vi "second gate increment fake.vi"(10 "Increment":dbl, 11 "Gate Voltage":dbl) -> ()   [LabVIEW 2021]
panel:
  in  "Voltage Safety Limit":dbl
  # "Second Gate\n Increment"
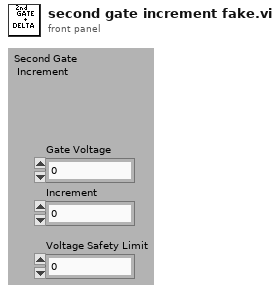
[diagram p1: front panel]
types:
  T1 = enum16{"Set Voltage", "Read Voltage", "Read Current", "Output On", "Output Off"}
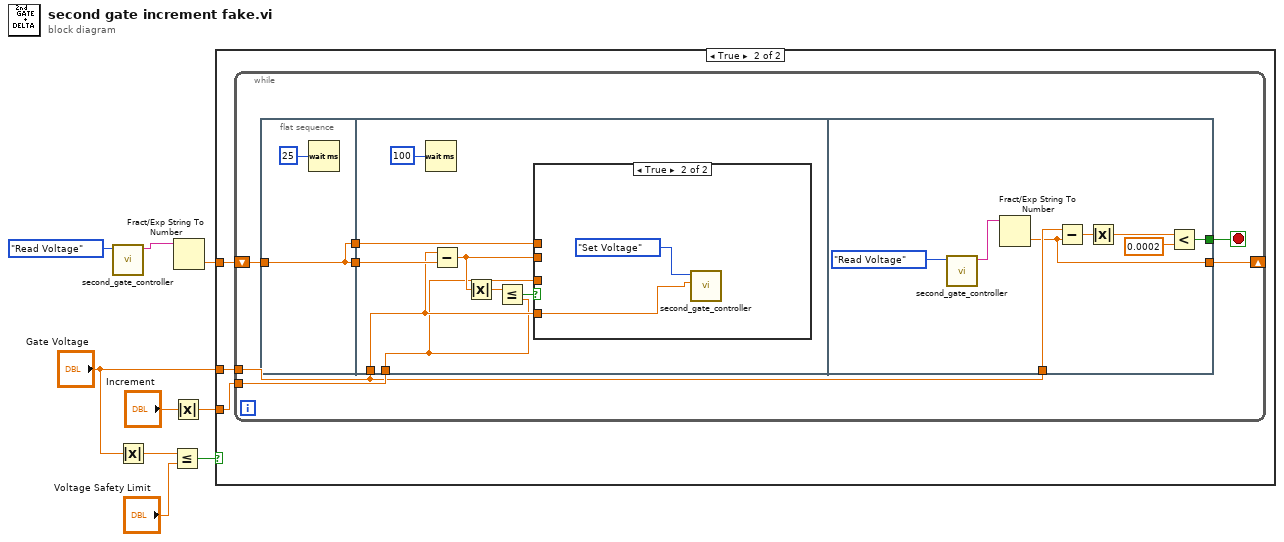
[diagram p0: block diagram]
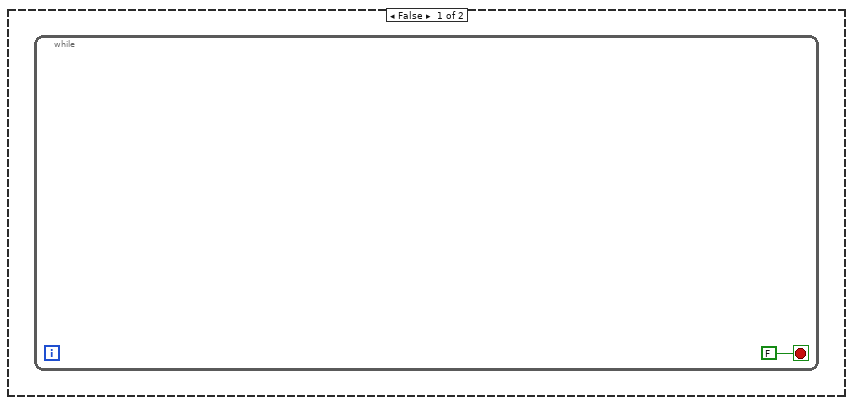
[diagram p2: hidden frame]
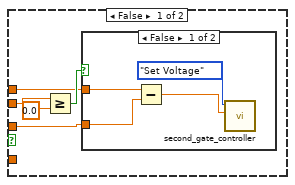
[diagram p3: hidden frame]
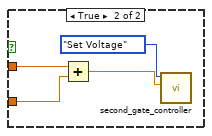
[diagram p4: hidden frame]
diagram:
  n1 = call "second_gate_controller.vi"("Command"=T1."Read Voltage") -> ("Response"=w2:string)  [unwired: 10 in]
  n2 = Absolute Value(x="Gate Voltage") -> (abs(x)=w7:dbl)
  n3 = Less Or Equal?(x=w7, y="Voltage Safety Limit") -> (x <= y?=w6:bool)
  n4 = Absolute Value(x="Increment") -> (abs(x)=w8:dbl)
  n5 = Fract/Exp String To Number(string=w2) -> (number=w9:dbl)  [unwired: 3 in, 1 out]
  n6 = case shown="True" w6 {
    tunnel: "Gate Voltage" -> [_ w13]
    tunnel: w9 -> [_ w12]
    tunnel: w8 -> [_ w11]
    frame False {
      n7 = while {
        stop <- FALSE stop-if-true
      }
    }
    frame True {
      n8 = while {
        tunnel: w13 -> [w18]
        tunnel: w11 -> [w19]
        shift-right: [w14] -> _
        shift-left: w12 -> [w15]
        stop <- w17 stop-if-true
        n9 = flat-sequence {
          tunnel: [w21] -> w20
          tunnel: [w21] -> w16
          tunnel: w15 -> [w21]
          tunnel: w18 -> [w27]
          tunnel: w20 -> [w30]
          tunnel: w19 -> [w24]
          tunnel: w16 -> [w23]
          tunnel: w18 -> [w53]
          tunnel: [w49] -> w17
          tunnel: [w48] -> w14
          frame #0 {
            n10 = Wait (ms)(milliseconds to wait=u32 25) -> ()  [unwired: 1 out]
          }
          frame #1 {
            n11 = Wait (ms)(milliseconds to wait=u32 100) -> ()  [unwired: 1 out]
            n12 = Subtract(x=w27, y=w30) -> (x-y=w25:dbl)
            n13 = Absolute Value(x=w25) -> (abs(x)=w29:dbl)
            n14 = Less Or Equal?(x=w29, y=w24) -> (x <= y?=w28:bool)
            n15 = case shown="True" w28 {
              tunnel: w27 -> [_ w45]
              tunnel: w25 -> [w32 _]
              tunnel: w24 -> [w35 _]
              tunnel: w23 -> [w31 _]
              frame False {
                n16 = Greater Or Equal?(x=w32, y=0.0) -> (x >= y?=w34:bool)
                n17 = case shown="False" w34 {
                  tunnel: w35 -> [w39 w43]
                  tunnel: w31 -> [w38 w42]
                  frame False {
                    n18 = Subtract(x=w38, y=w39) -> (x-y=w37:dbl)
                    n19 = call "second_gate_controller.vi"("Numerical Argument"=w37, "Command"=T1."Set Voltage") -> ()  [unwired: 9 in, 1 out]
                  }
                  frame True {
                    n20 = Add(x=w42, y=w43) -> (x+y=w41:dbl)
                    n21 = call "second_gate_controller.vi"("Numerical Argument"=w41, "Command"=T1."Set Voltage") -> ()  [unwired: 9 in, 1 out]
                  }
                }
              }
              frame True {
                n22 = call "second_gate_controller.vi"("Numerical Argument"=w45, "Command"=T1."Set Voltage") -> ()  [unwired: 9 in, 1 out]
              }
            }
          }
          frame #2 {
            n23 = call "second_gate_controller.vi"("Command"=T1."Read Voltage") -> ("Response"=w46:string)  [unwired: 10 in]
            n24 = Fract/Exp String To Number(string=w46) -> (number=w48:dbl)  [unwired: 3 in, 1 out]
            n25 = Subtract(x=w53, y=w48) -> (x-y=w52:dbl)
            n26 = Absolute Value(x=w52) -> (abs(x)=w51:dbl)
            n27 = Less?(x=w51, y=0.0002) -> (x < y?=w49:bool)
          }
        }
      }
    }
  }
